vi "stopAddingToBuffer.vi"(8 "error in (no error)":errorcluster, 11 "ElectrometerController in":refnum<class "ElectrometerController.lvclass">) -> (0 "error out":errorcluster, 3 "ElectrometerController out":refnum<class "ElectrometerController.lvclass">)   [LabVIEW 2016, in "ElectrometerController.lvclass"]
uses:
  ElectrometerController.lvclass
  Electrometer/Electrometer.lvclass
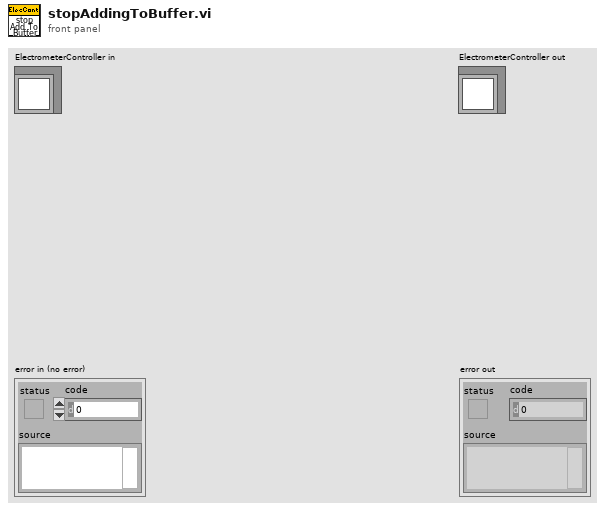
[diagram p1: front panel]
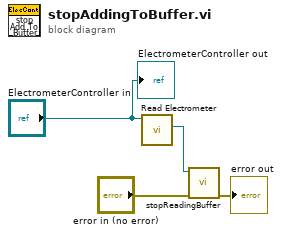
[diagram p0: block diagram]
diagram:
  n1 = call-dynamic "Read Electrometer.vi"("ElectrometerController in"="ElectrometerController in") -> ("Electrometer.lvclass"=w3:refnum<class "Electrometer.lvclass">)  [unwired: 8 in, 2 out]
  n2 = call "stopReadingBuffer.vi"("error in (no error)"="error in (no error)", "Electrometer in"=w3) -> ("error out"=→"error out":errorcluster)  [unwired: 8 in, 1 out]
  "ElectrometerController out" <- "ElectrometerController in"
